vi "AFG3352X.configure.vi"(0 "i ref in":refnum<vi>, 2 "configureData":string[](array[string]), 3 "ms timeout (10000)":i32=10000, 5 "error in (no error)":errorcluster) -> (14 "i ref out":refnum<vi>, 17 "timed out":bool, 19 "error out":errorcluster)   [LabVIEW 2014, in "AFG3352X.lvlib"]
doc: "Opens the interface and configures the device."
uses:
  AFG3352X.lvlib
  CS_Core/CSApplicationBaseClasses/AFGBase/AFGBase.waveformType.ctl
  CSlibraries/UtilityLib/UtilityLib.valueStatus.ctl
  CS_Core/CSApplicationBaseClasses/DeviceBase/DeviceBase.lvlib
  CS_Core/CSApplicationBaseClasses/AFGBase/AFGBase.lvlib
  CSlibraries/UtilityLib/UtilityLib.lvlib
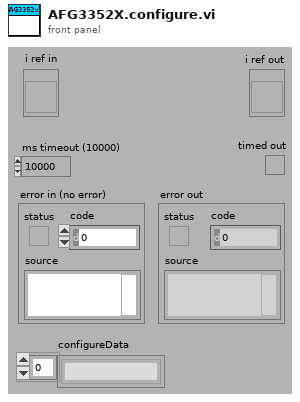
[diagram p1: front panel]
types:
  T1 = typedef "UtilityLib.lvlib/UtilityLib.valueStatus.ctl" = enum16{"no info available", "stand by/off", "on", "warning", "alarm/malfunction", "not implemented", "user action required", "important information", "system default", "control default", "indicator default", "button default"}
  T2 = typedef "AFGBase.lvlib/AFGBase.waveformType.ctl" = enum16{"sine", "square", "ramp", "pulse", "noise", "DC", "arbitrary", "triangle", "ramp_up", "ramp_down", "amplitude modulation"}
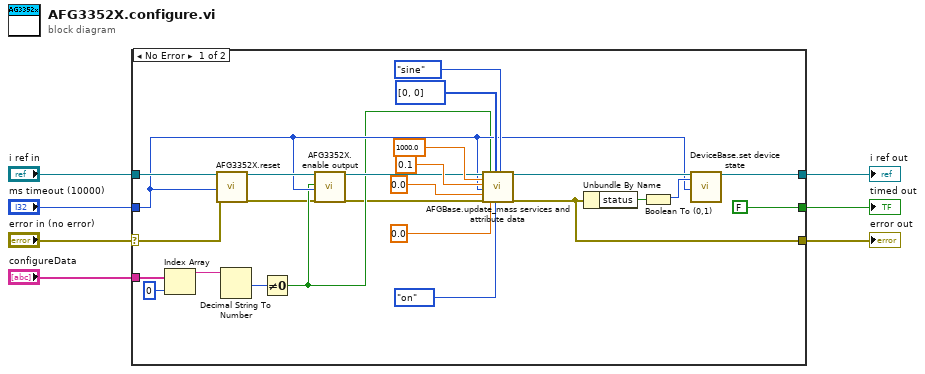
[diagram p0: block diagram]
diagram:
  n1 = case shown="No Error" "error in (no error)" {
    selector: "error in (no error)" -> [w14 w33]
    tunnel: [FALSE _] -> w7
    tunnel: [w29 w34] -> w6
    tunnel: "ms timeout (10000)" -> [w11 _]
    tunnel: "i ref in" -> [w15 w34]
    tunnel: [w27 w33] -> w2
    tunnel: "configureData" -> [w19 _]
    frame No Error {
      n2 = Index Array(array=w19, index=0) -> (element=w17:string)
      n3 = call "AFG3352X.reset.vi"("i ref in"=w15, "ms timeout (10000)"=w11, "error in (no error)"=w14) -> ("i ref out"=w13:refnum<vi>, "error out"=w9:errorcluster)  [unwired: 14 in, 1 out]
      n4 = Decimal String To Number(string=w17) -> (number=w16:i32)  [unwired: 2 in, 1 out]
      n5 = Not Equal To 0?(x=w16) -> (x != 0?=w10:bool)
      n6 = call "AFG3352X.enable output.vi"("i ref in"=w13, "outputEnable"=w10, "ms timeout (10000)"=w11, "error in (no error)"=w9) -> ("i ref out"=w12:refnum<vi>, "error out"=w8:errorcluster)  [unwired: 13 in, 1 out]
      n7 = call "AFGBase.update_mass services and attribute data.vi"("i ref in"=w12, "frequency"=1000.0, "amplitude"=0.1, "ms timeout (10000)"=w11, "phase"=0.0, "error in (no error)"=w8, "enableOutput"=w10, "DCOffset"=0.0, "trigger"=i16[] [0, 0], "valueStatus"=UtilityLib.valueStatus."on", "waveformType"=AFGBase.waveformType."sine") -> ("i ref out"=w28:refnum<vi>, "error out"=w27:errorcluster)  [unwired: 6 in, 1 out]
      n8 = Unbundle By Name(w27) -> ("status"=w30:bool)
      n9 = Boolean To (0,1)(Boolean=w30) -> (0, 1=w31:i16)
      n10 = call "DeviceBase.set device state.vi"("i ref in"=w28, "deviceState"=w31, "ms timeout (10000)"=w11) -> ("i ref out"=w29:refnum<vi>)  [unwired: 14 in, 2 out]
    }
    frame Error {
    }
  }
  "error out" <- w2
  "i ref out" <- w6
  "timed out" <- w7
